vi "LOGIC_GetNumberFromName.vi"(8 "error in (no error)":errorcluster, 11 "Database RefNum in":T1) -> (0 "error out":errorcluster, 1 "lastimg":string, 2 "number":i32)   [LabVIEW 2016]
uses:
  DBSHAND/private/vis/DatabaseHand_RefNum.ctl
  DBSHAND/private/vis/DatabaseHand_Element_Get(string).vi
  DBSHAND/private/vis/DatabaseHand_Element_Get(I32).vi
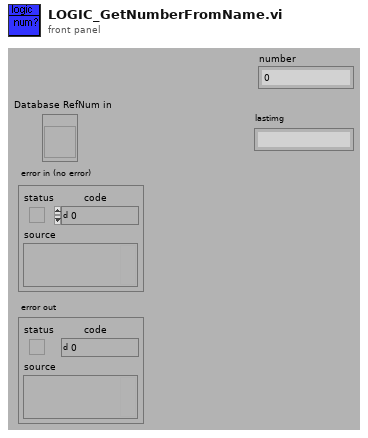
[diagram p1: front panel]
types:
  T1 = typedef "DatabaseHand_RefNum.ctl" = refnum<vi>
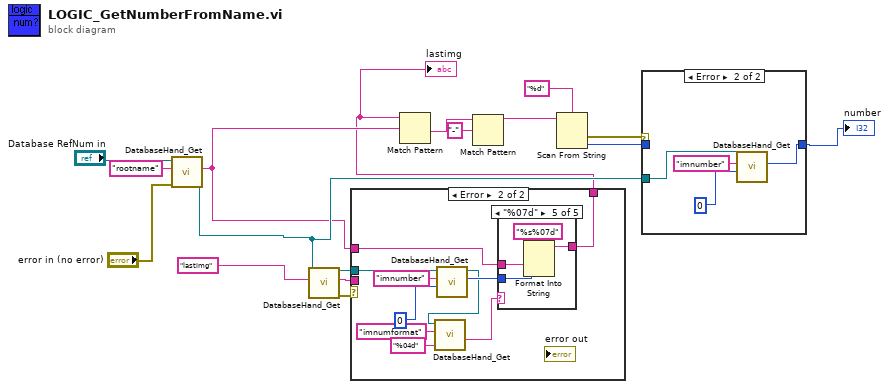
[diagram p0: block diagram]
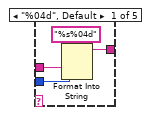
[diagram p4: hidden frame]
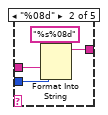
[diagram p5: hidden frame]
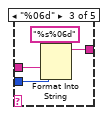
[diagram p6: hidden frame]
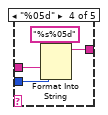
[diagram p7: hidden frame]
diagram:
  n1 = call-poly "DatabaseHand_Get.vi"("error in (no error)"="error in (no error)", "name"="rootname", "Database RefNum in"="Database RefNum in") -> ("value"=w3:string, "Database RefNum out"=w5:T1)  [unwired: 2 in, 5 out]
  n2 = call-poly "DatabaseHand_Get.vi"("name"="lastimg", "Database RefNum in"=w5) -> ("error out"=w14:errorcluster, "value"=w12:string, "Database RefNum out"=w13:T1)  [unwired: 3 in, 4 out]
  n3 = case shown="Error" w14 {
    tunnel: w13 -> [_ w28]
    tunnel: w3 -> [_ w25]
    tunnel: [w18 w23] -> w1
    tunnel: w12 -> [w18 _]
    frame No Error {
    }
    frame Error {
      n4 = call-poly "DatabaseHand_Get.vi"("default value"=0 ("number"), "name"="imnumber", "Database RefNum in"=w28) -> ("value"=w24:i32, "Database RefNum out"=w22:T1)  [unwired: 2 in, 5 out]
      n5 = call-poly "DatabaseHand_Get.vi"("default value"="%04d", "name"="imnumformat", "Database RefNum in"=w22) -> ("type"=w19:string)  [unwired: 2 in, 6 out]
      n6 = case shown="\"%07d\"" w19 {
        tunnel: w25 -> [w32 w36 w40 w44 w48]
        tunnel: w24 -> [w31 w35 w39 w43 w47]
        tunnel: [w29 w33 w37 w41 w45] -> w23
        frame "%04d", Default {
          n7 = Format Into String(format string="%s%04d", w32, w31) -> (resulting string=w29:string)  [unwired: 2 in, 1 out]
        }
        frame "%08d" {
          n8 = Format Into String(format string="%s%08d", w36, w35) -> (resulting string=w33:string)  [unwired: 2 in, 1 out]
        }
        frame "%06d" {
          n9 = Format Into String(format string="%s%06d", w40, w39) -> (resulting string=w37:string)  [unwired: 2 in, 1 out]
        }
        frame "%05d" {
          n10 = Format Into String(format string="%s%05d", w44, w43) -> (resulting string=w41:string)  [unwired: 2 in, 1 out]
        }
        frame "%07d" {
          n11 = Format Into String(format string="%s%07d", w48, w47) -> (resulting string=w45:string)  [unwired: 2 in, 1 out]
        }
      }
    }
  }
  "lastimg" <- w1
  n12 = Match Pattern(string=w1, regular expression=w3) -> (after substring=w11:string)  [unwired: 4 out]
  n13 = Match Pattern(string=w11, regular expression="-") -> (before substring=w9:string)  [unwired: 4 out]
  n14 = Scan From String(format string="%d", input string=w9) -> (error out=w7:errorcluster, output 1=w6:i32)  [unwired: 2 in, 3 out]
  n15 = case shown="Error" w7 {
    tunnel: w6 -> [w49 _]
    tunnel: w5 -> [_ w51]
    tunnel: [w49 w50] -> w4
    frame No Error {
    }
    frame Error {
      n16 = call-poly "DatabaseHand_Get.vi"("default value"=0 ("number"), "name"="imnumber", "Database RefNum in"=w51) -> ("value"=w50:i32)  [unwired: 2 in, 6 out]
    }
  }
  "number" <- w4
